vi "Close.vi"(8 "error in (no error)":errorcluster, 11 "VISA resource name":refnum<visa-resource-name>) -> (0 "error out":errorcluster)   [LabVIEW 2012, in "Surelite I.lvlib"]
doc: "Performs an instrument error query before terminating the software connection to the instrument."
uses:
  Surelite I.lvlib
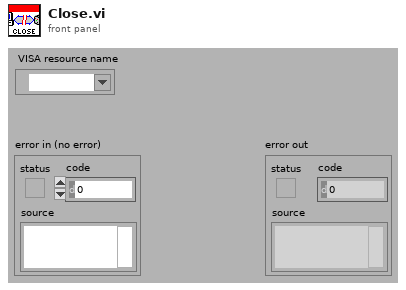
[diagram p1: front panel]
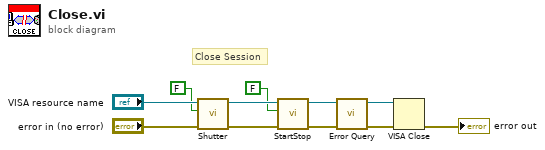
[diagram p0: block diagram]
diagram:
  # "Close Session"
  n1 = call "Shutter.vi"("Open? (F)"=FALSE, "VISA resource name"="VISA resource name") -> ("VISA resource name out"=w3:refnum<visa-resource-name>)  [unwired: 8 in, 1 out]
  n2 = call "StartStop.vi"("Start? (F)"=FALSE, "VISA resource name"=w3) -> ("VISA resource name out"=w4:refnum<visa-resource-name>)  [unwired: 8 in, 1 out]
  n3 = call "Error Query.vi"("error in (no error)"="error in (no error)", "VISA resource name"=w4) -> ("error out"=w6:errorcluster, "VISA resource name out"=w5:refnum<visa-resource-name>)  [unwired: 6 in, 2 out]
  n4 = VISA Close(VISA resource name=w5, error in (no error)=w6) -> (error out=→"error out":errorcluster)
